vi "modbus slave new.vi"() -> ()   [LabVIEW 2016]
uses:
  <vilib>/NI/Modbus Library/API/Wrapper/Create TCP Slave.vi
  <vilib>/NI/Modbus Library/API/slave/Modbus Slave.lvclass
  <vilib>/NI/Modbus Library/API/Wrapper/API Main.lvlib
  <vilib>/ptbypt/NI_PtbyPt.lvlib
  <vilib>/Utility/config.llb/NI_LVConfig.lvlib
panel:
  out "读取register values 2":u16[](array[numeric])
  out "status":bool
  in  "写入registers to write":u16[](array[numeric])
  out "读取register values":u16[](array[numeric])
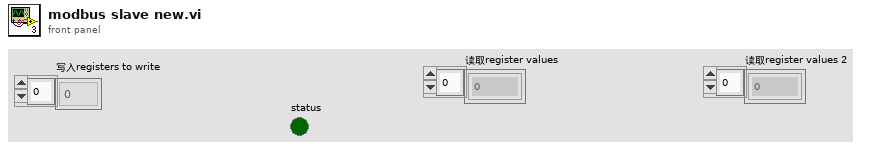
[diagram p1: front panel]
types:
  T1 = enum16{"启动整机", "停止整机", "标样核查", "加标回收", "平行样测试", "零点核查", "跨度核查", "校零", "校标"}
  T2 = cluster{"status":bool, "代码":u16, "source":string}
  T3 = cluster{"COD浓度（mg/L)":dbl, "水样启动时间":timestamp, "加标回收启动时间":timestamp, "CODMn工作状态":enum16{"空闲", "水样测试", "标样核查", "零点核查", "跨度核查", "空白测试", "平行样测试", "加标回收", "空白校准", "标样校准", "初始化（清洗）"}, "多列列表框":i32}
  T4 = cluster{"系统时间":timestamp, "工作状态":enum16{"空闲", "水样测试", "标样核查", "零点核查", "跨度核查", "空白测试", "平行样测试", "加标回收", "空白校准", "标样校准", "初始化（清洗）"}, "测量模式":enum16{"待机", "连续模式", "周期模式", "定点模式", "受控模式", "手动模式"}, "告警代码":u16, "故障代码":u16, "日志代码":u16, "软件版本":u16, "F0":sgl, "F1":sgl, "F2":sgl, "F3":sgl, "T":sgl, "H":sgl, "id":u16, "flowid":u16, "量程":u16, "总磷控温温度1":sgl, "营养盐控温温度2":sgl, "ADC":sgl}
  T5 = enum16{"空闲", "水样测试", "标样核查", "零点核查", "跨度核查", "空白测试", "平行样测试", "加标回收", "空白校准", "标样校准", "初始化（清洗）"}
  T6 = typedef "NI_LVConfig.lvlib/Config Data RefNum.ctl" = refnum<k1>
  T7 = enum16{"", "CODMn", "PH", "氨氮", "总氮", "总磷", "CODCr", "电导率", "水温", "溶解氧", "浊度", "叶绿素", "藻密度", "ORP"}
  T8 = enum16{"i13001", "i13002", "i13003", "i13004", "i13005", "i13006", "i13007", "i13008", "i13009", "i13010", "i13011", "i13012", "i13013", "i13014", "i13015", "i13016", "i13017", "i13101", "i13102", "i13103", "i13104", "i13105", "i13106", "i13107", "i13108", "i13109", "i13110"}
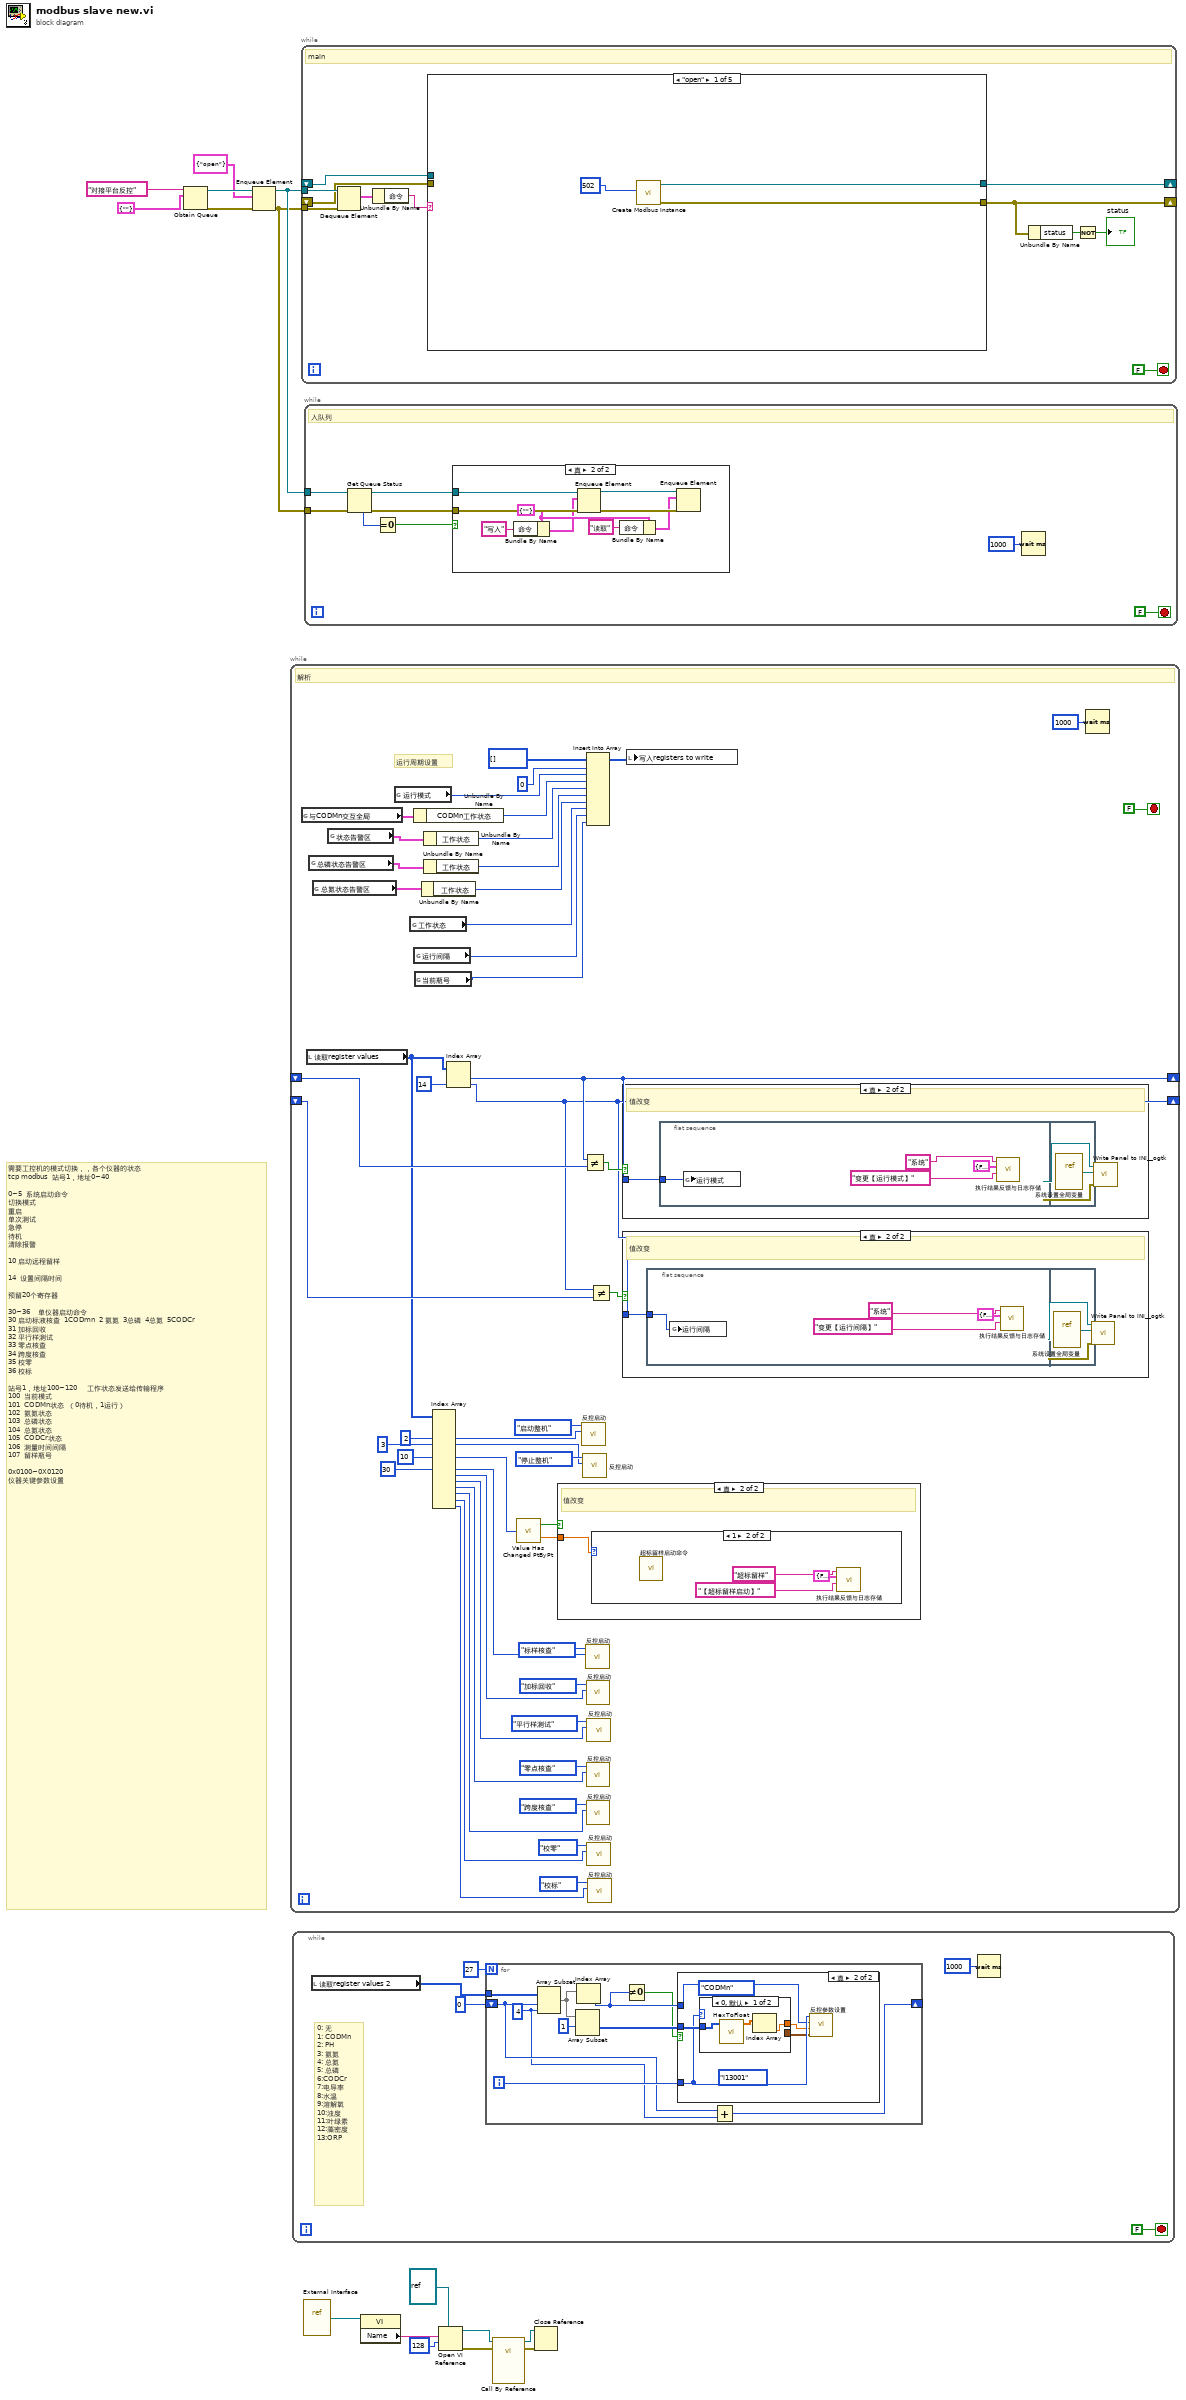
[diagram p0: block diagram]
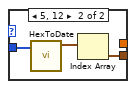
[diagram p3: hidden frame]
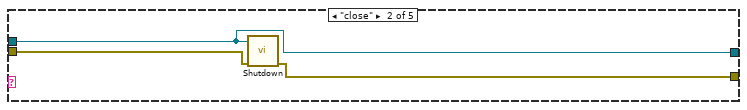
[diagram p9: hidden frame]
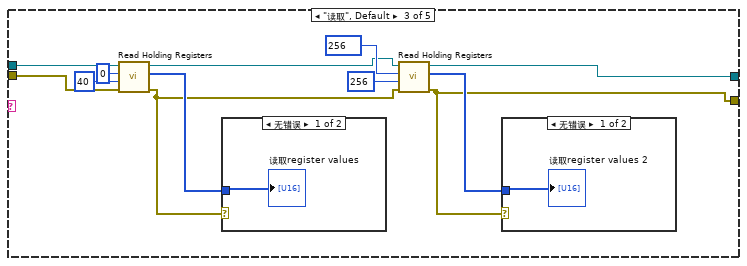
[diagram p10: hidden frame]
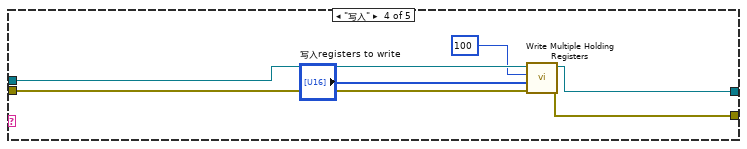
[diagram p13: hidden frame]
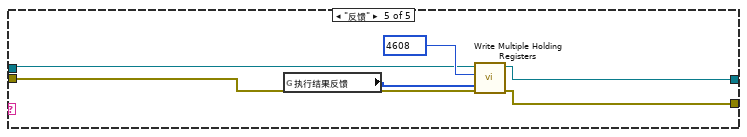
[diagram p14: hidden frame]
diagram:
  # "需要工控机的模式切换，，各个仪器的状态\ntcp modbus  站号1，地址0~40\n\n0~5  系统启动命令\n切换模式\n重启\n单次测试\n急停\n待机\n清除报警\n\n10 启动远程留样\n\n14  设置间隔时间\n\n预留20个寄存器\n\n30~36    单仪器启动命令\n30 启动标液核查  1CODmn  2 氨氮  3总磷  4总氮  5CODCr\n31 加标回收\n32 平行样测试\n33 零点核查\n34 跨度核查\n35 校零\n36 校标\n\n站号1，地址100~120     工作状态发送给传输程序\n100  当前模式\n101  CODMn状态  （0待机，1运行）\n102  氨氮状态\n103  总磷状态\n104  总氮状态\n105  CODCr状态\n106  测量时间间隔\n107  留样瓶号\n\n0x0100~0X0120\n仪器关键参数设置"
  n1 = Obtain Queue(name (unnamed)="对接平台反控" ("名称（未命名）"), element data type=cluster{"命令":string} {"命令"=""}) -> (queue out=w13:refnum<queue>, error out=w12:errorcluster)  [unwired: 3 in, 1 out]
  n2 = Enqueue Element(queue=w13, element=cluster{"命令":string} {"命令"="open"} ("元素"), error in (no error)=w12) -> (queue out=w10:refnum<queue>, error out=w9:errorcluster)  [unwired: 1 in, 1 out]
  n3 = while {
    shift-right: [w51] -> _
    shift-left: _ -> [w53]
    shift-right: [w48] -> _
    shift-left: _ -> [w50]
    stop <- FALSE stop-if-true
    # "运行周期设置"
    # "解析"
    n4 = global read "modbus slave全局.vi" "与CODMn交互全局"() -> (w20:T3)
    n5 = local read "读取register values"() -> (w43:u16[])
    n6 = global read "VAR总磷总氮全局变量.vi" "总磷状态告警区"() -> (w17:T4)
    n7 = global read "VAR总磷总氮全局变量.vi" "总氮状态告警区"() -> (w16:T4)
    n8 = global read "VAR总磷总氮全局变量.vi" "状态告警区"() -> (w18:T4)
    n9 = global read "系统设置全局变量.vi" "运行模式"() -> (w62:enum16{"维护模式", "常规模式", "应急模式", "质控模式"})
    n10 = global read "CODcr全局变量.vi" "工作状态"() -> (w57:T5)
    n11 = Unbundle By Name(w20) -> ("CODMn工作状态"=w19:T5)
    n12 = global read "系统设置全局变量.vi" "运行间隔"() -> (w56:i16)
    n13 = global read "外部交互全局.vi" "当前瓶号"() -> (w21:u16)
    n14 = Unbundle By Name(w16) -> ("工作状态"=w58:T5)
    n15 = Unbundle By Name(w18) -> ("工作状态"=w60:T5)
    n16 = Unbundle By Name(w17) -> ("工作状态"=w59:T5)
    n17 = Index Array(array=w43, index #3=2 ("索引"), index #4=3 ("索引"), index #6=10 ("索引"), index #8=30 ("索引")) -> (element #3=w42:u16, element #4=w39:u16, element #6=w36:u16, element #8=w34:u16, element #9=w28:u16, element #10=w27:u16, element #11=w26:u16, element #12=w24:u16, element #13=w23:u16, element #14=w22:u16)  [unwired: 10 in, 4 out]
    n18 = Index Array(array=w43, index #2=14 ("索引")) -> (element #1=w51:u16, element #2=w48:u16)  [unwired: 1 in]
    n19 = call <vilib>:"Value Has Changed PtByPt.vi"("input data point"=w36) -> ("has changed"=w38:bool, "output data point"=w37:dbl)  [unwired: 1 in]
    n20 = case shown="真" w38 {
      tunnel: w37 -> [_ w66]
      frame False {
      }
      frame True {
        # "值改变"
        n21 = case shown="1" w66 {
          frame 0, Default {
          }
          frame 1 {
            n22 = call "超标留样启动命令.vi"() -> ()  [unwired: 12 in]
            n23 = call "执行结果反馈与日志存储.vi"("日志信息"="【超标留样启动】", "error out"=T2 {"status"=FALSE, "代码"=1, "source"=""}, "设备"="超标留样") -> ()  [unwired: 9 in]
          }
        }
      }
    }
    n24 = call "反控启动.vi"("启动参数"=w42, "启动类型"=T1."启动整机") -> ()  [unwired: 10 in]
    n25 = call "反控启动.vi"("启动参数"=w39, "启动类型"=T1."停止整机") -> ()  [unwired: 10 in]
    n26 = Not Equal?(x=w51, y=w53) -> (x != y?=w52:bool)
    n27 = call "反控启动.vi"("启动参数"=w34, "启动类型"=T1."标样核查") -> ()  [unwired: 10 in]
    n28 = Insert Into Array(array=u16[] [] ("values to write"), index=0 ("索引"), new element #1=w62, new element #2=w19, new element #3=w60, new element #4=w59, new element #5=w58, new element #6=w57, new element #7=w56, new element #8=w21) -> (w55:u16[])
    n29 = call "反控启动.vi"("启动参数"=w28, "启动类型"=T1."加标回收") -> ()  [unwired: 10 in]
    n30 = call "反控启动.vi"("启动参数"=w26, "启动类型"=T1."零点核查") -> ()  [unwired: 10 in]
    n31 = call "反控启动.vi"("启动参数"=w24, "启动类型"=T1."跨度核查") -> ()  [unwired: 10 in]
    n32 = call "反控启动.vi"("启动参数"=w27, "启动类型"=T1."平行样测试") -> ()  [unwired: 10 in]
    n33 = call "反控启动.vi"("启动参数"=w23, "启动类型"=T1."校零") -> ()  [unwired: 10 in]
    n34 = call "反控启动.vi"("启动参数"=w22, "启动类型"=T1."校标") -> ()  [unwired: 10 in]
    n35 = Not Equal?(x=w48, y=w50) -> (x != y?=w49:bool)
    n36 = case shown="真" w52 {
      tunnel: w51 -> [_ w89]
      frame False {
      }
      frame True {
        # "值改变"
        n37 = flat-sequence {
          tunnel: w89 -> [w93]
          frame #0 {
            n38 = global write "系统设置全局变量.vi" "运行模式"(w93) -> ()
            n39 = call "执行结果反馈与日志存储.vi"("日志信息"="变更【运行模式】", "error out"=T2 {"status"=FALSE, "代码"=1, "source"=""}, "设备"="系统") -> ()  [unwired: 9 in]
          }
          frame #1 {
            n40 = call <vilib>:"Application Directory.vi"() -> ("Application Directory"=w107:path)
            n41 = Build Path(base path=w107, name or relative path="data\\sys.ini" ("名称或相对路径")) -> (appended path=w105:path)
            n42 = call <vilib>:"Open Config Data.vi"("configuration file path"=w105) -> ("error out"=w101:errorcluster, "refnum"=w104:T6)  [unwired: 8 in, 1 out]
            n43 = vi-ref "系统设置全局变量.vi"() -> (w103:refnum<vi>)
            n44 = call <userlib>:"Write Panel to INI__ogtk.vi"("error in (no error)"=w101, "VI ref"=w103, "refnum"=w104) -> ("error out"=w100:errorcluster, "refnum out"=w102:T6)  [unwired: 7 in]
            n45 = call <vilib>:"Close Config Data.vi"("error in (no error)"=w100, "refnum"=w102) -> ("error out"=w95:errorcluster, "file path"=w94:path)  [unwired: 8 in]
            n46 = Open/Create/Replace File(file path (use dialog)=w94, error in=w95) -> (refnum out=w98:refnum<file>, error out=w99:errorcluster)  [unwired: 4 in, 1 out]
            n47 = Flush File(refnum=w98, error in=w99) -> (refnum out=w97:refnum<file>, error out=w96:errorcluster)
            n48 = Close File(refnum=w97, error in=w96) -> ()  [unwired: 2 out]
          }
        }
      }
    }
    n49 = case shown="真" w49 {
      tunnel: w48 -> [_ w70]
      frame False {
      }
      frame True {
        # "值改变"
        n50 = flat-sequence {
          tunnel: w70 -> [w74]
          frame #0 {
            n51 = global write "系统设置全局变量.vi" "运行间隔"(w74) -> ()
            n52 = call "执行结果反馈与日志存储.vi"("日志信息"="变更【运行间隔】", "error out"=T2 {"status"=FALSE, "代码"=1, "source"=""}, "设备"="系统") -> ()  [unwired: 9 in]
          }
          frame #1 {
            n53 = call <vilib>:"Application Directory.vi"() -> ("Application Directory"=w88:path)
            n54 = Build Path(base path=w88, name or relative path="data\\sys.ini" ("名称或相对路径")) -> (appended path=w86:path)
            n55 = call <vilib>:"Open Config Data.vi"("configuration file path"=w86) -> ("error out"=w82:errorcluster, "refnum"=w85:T6)  [unwired: 8 in, 1 out]
            n56 = vi-ref "系统设置全局变量.vi"() -> (w84:refnum<vi>)
            n57 = call <userlib>:"Write Panel to INI__ogtk.vi"("error in (no error)"=w82, "VI ref"=w84, "refnum"=w85) -> ("error out"=w81:errorcluster, "refnum out"=w83:T6)  [unwired: 7 in]
            n58 = call <vilib>:"Close Config Data.vi"("error in (no error)"=w81, "refnum"=w83) -> ("error out"=w76:errorcluster, "file path"=w75:path)  [unwired: 8 in]
            n59 = Open/Create/Replace File(file path (use dialog)=w75, error in=w76) -> (refnum out=w79:refnum<file>, error out=w80:errorcluster)  [unwired: 4 in, 1 out]
            n60 = Flush File(refnum=w79, error in=w80) -> (refnum out=w78:refnum<file>, error out=w77:errorcluster)
            n61 = Close File(refnum=w78, error in=w77) -> ()  [unwired: 2 out]
          }
        }
      }
    }
    n62 = local write "写入registers to write"(w55) -> ()
    n63 = Wait (ms)(milliseconds to wait=u32 1000 ("等待时间（毫秒）")) -> ()  [unwired: 1 out]
  }
  n64 = while {
    stop <- FALSE stop-if-true
    # "0: 无\n1: CODMn\n2: PH\n3: 氨氮\n4: 总氮\n5: 总磷\n6:CODCr\n7:电导率\n8:水温\n9:溶解氧\n10:浊度\n11:叶绿素\n12:藻密度\n13:ORP"
    n65 = local read "读取register values 2"() -> (w110:u16[])
    n66 = for {
      N: 27 -> [_]
      tunnel: w110 -> [w122]
      shift-right: [w113] -> _
      shift-left: 0 ("索引") -> [w115]
      i -> [w118]
      w114 = 4 ("长度")
      n67 = Array Subset(array=w122, index=w115, length=w114) -> (w121:u16[])
      n68 = Array Subset(array=w121, index=1 ("索引")) -> (w119:u16[])  [unwired: 1 in]
      n69 = Index Array(array=w121) -> (element=w117:u16)  [unwired: 1 in]
      n70 = Not Equal To 0?(x=w117) -> (x != 0?=w116:bool)
      n71 = case shown="真" w116 {
        tunnel: w119 -> [_ w127]
        tunnel: w118 -> [_ w126]
        tunnel: w117 -> [_ w125]
        frame False {
        }
        frame True {
          (unwired) T7."CODMn"
          (unwired) T8."i13001" ("设置类型")
          n72 = case shown="0, 默认" w126 {
            tunnel: w127 -> [w129 w132]
            tunnel: [_ w133] -> w123
            tunnel: [w130 _] -> w124
            frame 0, Default {
              n73 = call "HexToFloat.vi"("数组"=w129) -> ("FLOAT"=w128:sgl[])  [unwired: 10 in]
              n74 = Index Array(array=w128) -> (element=w130:sgl)  [unwired: 1 in]
            }
            frame 5, 12 {
              n75 = call "HexToDate.vi"("数组"=w132) -> ("DATE"=w131:timestamp[])  [unwired: 10 in]
              n76 = Index Array(array=w131) -> (element=w133:timestamp)  [unwired: 1 in]
            }
          }
          n77 = call "反控参数设置.vi"("value time"=w123, "value float"=w124, "设置参数"=w125, "设置类型"=w126) -> ()  [unwired: 8 in]
        }
      }
      n78 = Add(x=w115, y=w114) -> (x+y=w113:i32)
    }
    n79 = Wait (ms)(milliseconds to wait=u32 1000 ("等待时间（毫秒）")) -> ()  [unwired: 1 out]
  }
  n80 = while {
    tunnel: w10 -> [w144]
    tunnel: w9 -> [w143]
    shift-right: [w140] -> _
    shift-left: _ -> [w139]
    shift-right: [w134] -> _
    shift-left: _ -> [w138]
    stop <- FALSE stop-if-true
    # "main"
    n81 = Dequeue Element(queue=w144, error in (no error)=w143) -> (element=w142:cluster{"命令":string})  [unwired: 1 in, 3 out]
    n82 = Unbundle By Name(w142) -> ("命令"=w141:string)
    n83 = case shown="\"open\"" w141 {
      tunnel: [w145 w148 w152 w166 w173] -> w140
      tunnel: [w146 w149 w151 w165 w172] -> w134
      tunnel: w139 -> [_ w148 w162 w170 w175]
      tunnel: w138 -> [_ w150 w161 w169 w174]
      frame "open" {
        n84 = call-poly <vilib>:"Create Modbus Instance.vi"("port (502)"=u16 502) -> ("error out"=w146:errorcluster, "TCP slave instance"=w145:refnum<class "Modbus Slave.lvclass">)  [unwired: 9 in]
      }
      frame "close" {
        n85 = call-dynamic "Shutdown.vi"("error in"=w150, "Modbus slave in"=w148) -> ("error out"=w149:errorcluster)  [unwired: 9 in]
      }
      frame "读取", Default {
        n86 = call-dynamic "Read Holding Registers.vi"("error in"=w161, "number of inputs"=u16 40, "starting address"=u16 0, "Modbus slave in"=w162) -> ("error out"=w153:errorcluster, "register values"=w158:u16[], "Modbus slave out"=w154:refnum<class "Modbus Slave.lvclass">)  [unwired: 5 in]
        n87 = case shown="无错误" w153 {
          tunnel: w158 -> [w164 _]
          frame No Error {
            "读取register values" <- w164
          }
          frame Error {
          }
        }
        n88 = call-dynamic "Read Holding Registers.vi"("error in"=w153, "number of inputs"=u16 256, "starting address"=u16 256, "Modbus slave in"=w154) -> ("error out"=w151:errorcluster, "register values"=w157:u16[], "Modbus slave out"=w152:refnum<class "Modbus Slave.lvclass">)  [unwired: 5 in]
        n89 = case shown="无错误" w151 {
          tunnel: w157 -> [w163 _]
          frame No Error {
            "读取register values 2" <- w163
          }
          frame Error {
          }
        }
      }
      frame "写入" {
        n90 = call-dynamic "Write Multiple Holding Registers.vi"("error in"=w169, "registers to write"="写入registers to write", "starting address"=u16 100, "Modbus slave in"=w170) -> ("error out"=w165:errorcluster, "Modbus slave out"=w166:refnum<class "Modbus Slave.lvclass">)  [unwired: 6 in]
      }
      frame "反馈" {
        n91 = global read "modbus slave全局.vi" "执行结果反馈"() -> (w171:u16[])
        n92 = call-dynamic "Write Multiple Holding Registers.vi"("error in"=w174, "registers to write"=w171, "starting address"=u16 4608, "Modbus slave in"=w175) -> ("error out"=w172:errorcluster, "Modbus slave out"=w173:refnum<class "Modbus Slave.lvclass">)  [unwired: 6 in]
      }
    }
    n93 = Unbundle By Name(w134) -> ("status"=w136:bool)
    n94 = Not(x=w136) -> (.not. x?=→"status":bool)
  }
  n95 = vi-ref "External Interface.vi"() -> (w8:refnum<vi>)
  n96 = while {
    tunnel: w10 -> [w184]
    tunnel: w9 -> [w182]
    stop <- FALSE stop-if-true
    # "入队列"
    n97 = Get Queue Status(queue=w184, error in (no error)=w182) -> (queue out=w183:refnum<queue>, error out=w181:errorcluster, # elements in queue=w180:i32)  [unwired: 1 in, 5 out]
    n98 = Equal To 0?(x=w180) -> (x = 0?=w179:bool)
    n99 = case shown="真" w179 {
      tunnel: w183 -> [_ w193]
      tunnel: w181 -> [_ w192]
      frame False {
      }
      frame True {
        w188 = cluster{"命令":string} {"命令"=""} ("元素")
        n100 = Bundle By Name(cluster=w188, "命令"="写入") -> (w187:cluster{"命令":string})
        n101 = Enqueue Element(queue=w193, element=w187, error in (no error)=w192) -> (queue out=w191:refnum<queue>, error out=w190:errorcluster)  [unwired: 1 in, 1 out]
        n102 = Bundle By Name(cluster=w188, "命令"="读取") -> (w185:cluster{"命令":string})
        n103 = Enqueue Element(queue=w191, element=w185, error in (no error)=w190) -> ()  [unwired: 1 in, 3 out]
      }
    }
    n104 = Wait (ms)(milliseconds to wait=u32 1000 ("等待时间（毫秒）")) -> ()  [unwired: 1 out]
  }
  n105 = property class="VI"(reference=w8) -> ("Name"=w7:string)  [unwired: 1 in, 2 out]
  n106 = Open VI Reference(type specifier VI Refnum (for type only)=refnum<vi> refnum, vi path=w7, options=128 ("选项")) -> (vi reference=w5:refnum<vi>, error out=w3:errorcluster)  [unwired: 3 in]
  n107 = call-by-ref "?"(reference=w5, error in=w3) -> (reference out=w1:refnum<vi>, error out=w2:errorcluster)  [unwired: 12 in]
  n108 = Close Reference(reference=w1, error in (no error)=w2) -> ()  [unwired: 1 out]
